vi "Test Sequence.vi"(0 "FeedBack Channel":string[](array[string])=["fgdgfvcbc", "vnfhgjkn", "21354682"], 1 "Test Name":string, 2 "Steps":T1(array[cluster]), 3 "Tracibility":bool) -> (6 "Emergency":bool, 7 "Out":i32, 8 "Condition":bool)   [LabVIEW 2015]
uses:
  <vilib>/Utility/error.llb/whitespace.ctl
  Galobal variable_TI.vi
  Project Setup/Globle Variable/GR_Servo.vi
  <vilib>/Instr/_visa.llb/VISA Configure Serial Port (Instr).vi
panel:
  out "error out 2":errorcluster
  out "error out":errorcluster
  out "Wait/Poll (ms)":u32
  out "Channels (Out)":i32[](array[numeric])
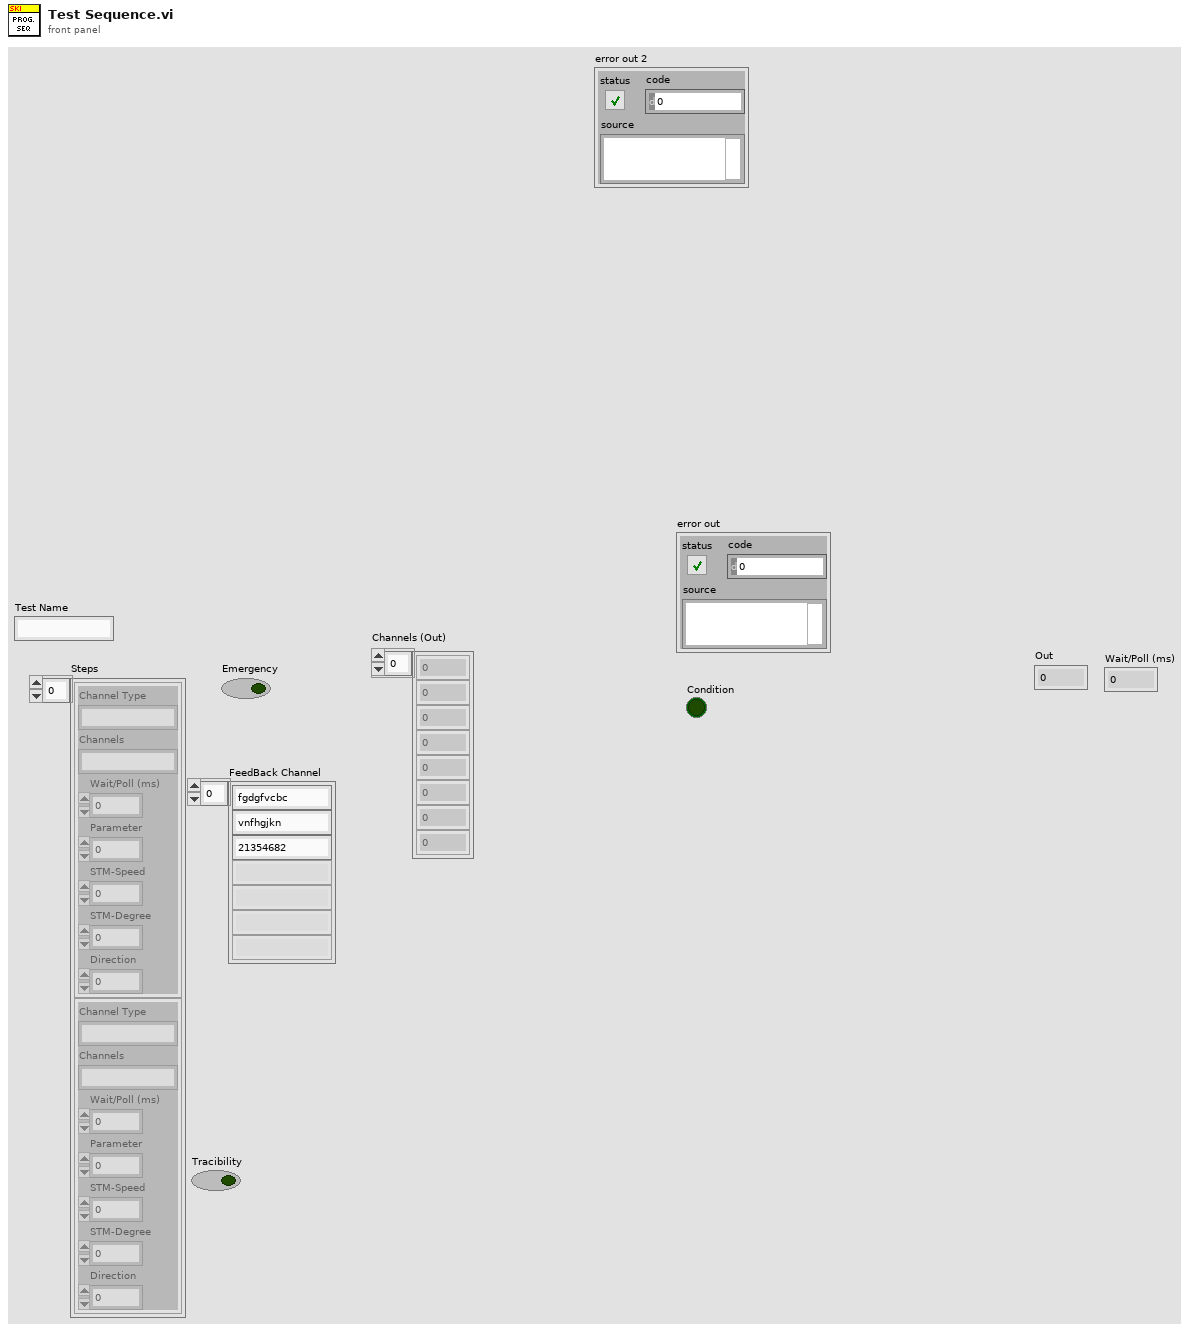
[diagram p1: front panel]
types:
  T1 = cluster{"Channel Type":string, "Channels":string, "Wait/Poll (ms)":u32, "Parameter":u8, "STM-Speed":i32, "STM-Degree":u32, "Direction":u8}[]
  T2 = cluster{"Emergency_1":bool, "Reset_2":bool, "Air Pressure_4":bool, "Safety Sensor_5":bool, "Safety Sensor_6":bool, "Barcode Rev rs_24":bool, "Clamp fwd rs_21":bool, "Servo Fault":bool, "Home _3":bool}
  T3 = cluster{"MIC ":refnum<visa-resource-name>, "baud rate MIC ":u32, "LCD ":refnum<visa-resource-name>, "baud rate_LCD":u32}
  T4 = cluster{"Model":string, "Difusser Code":string, "TFT Code ":string}
  T5 = typedef "whitespace.ctl" = u16
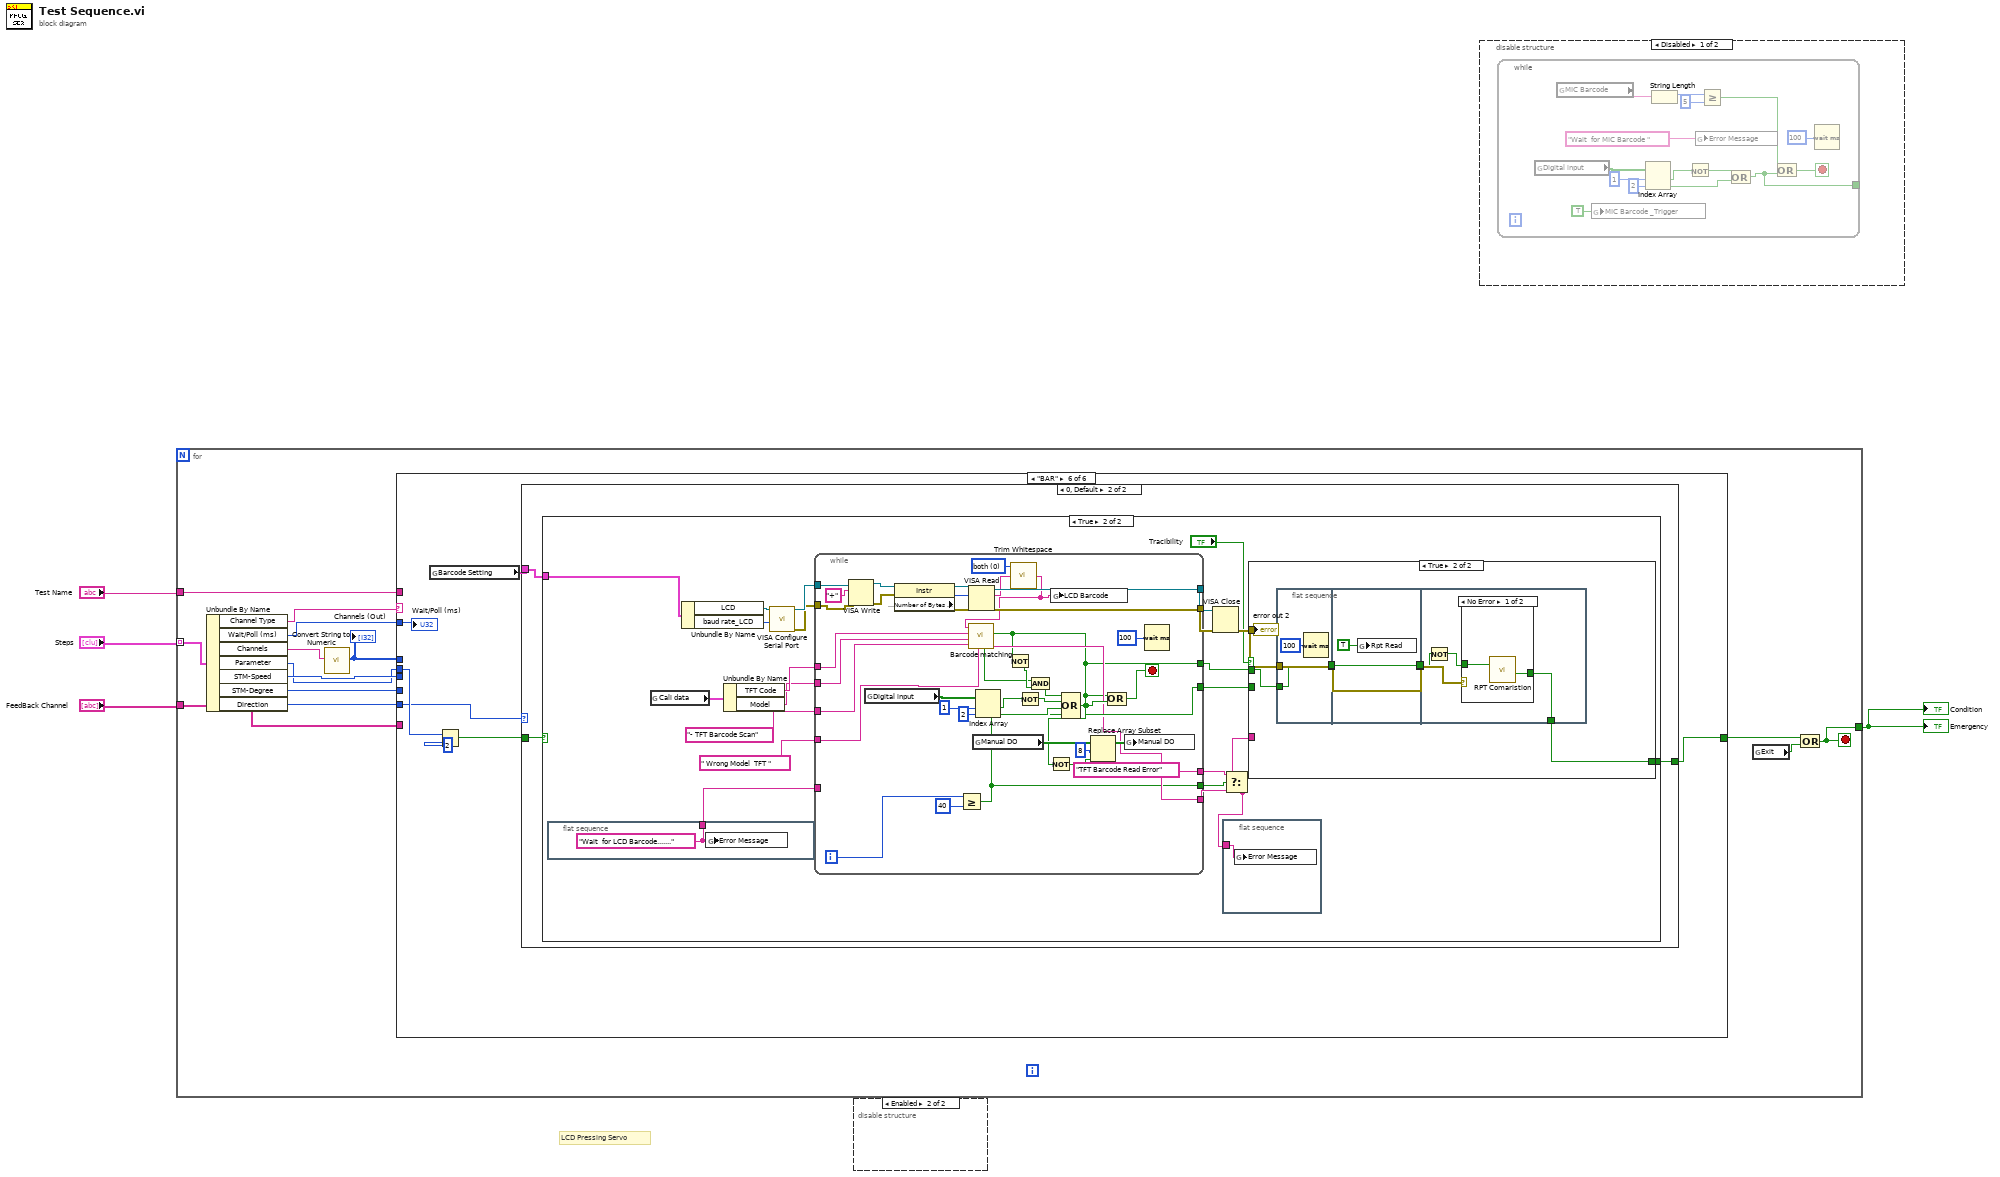
[diagram p0: block diagram]
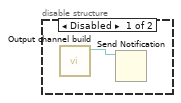
[diagram p3: hidden frame]
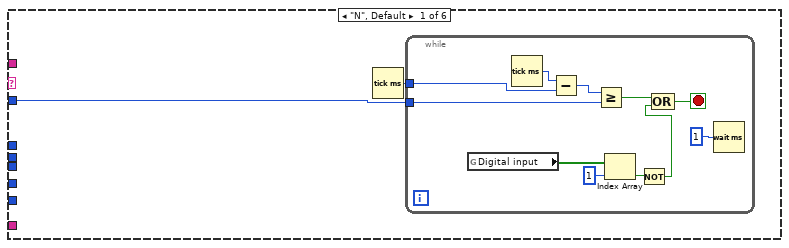
[diagram p4: hidden frame]
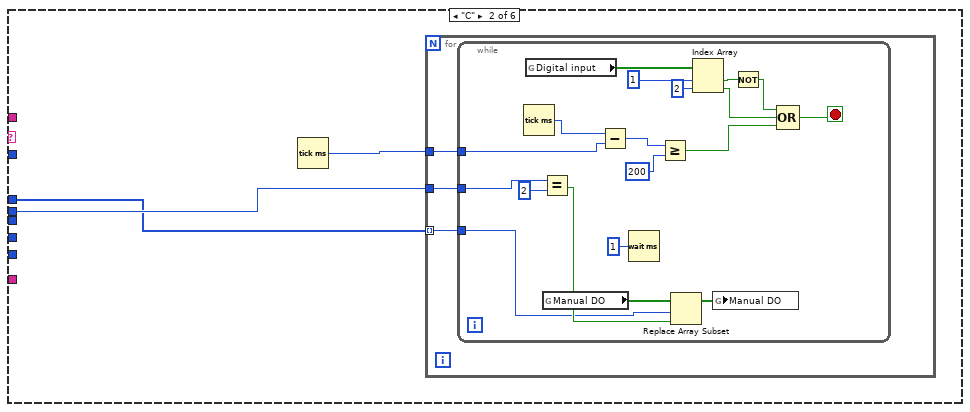
[diagram p5: hidden frame]
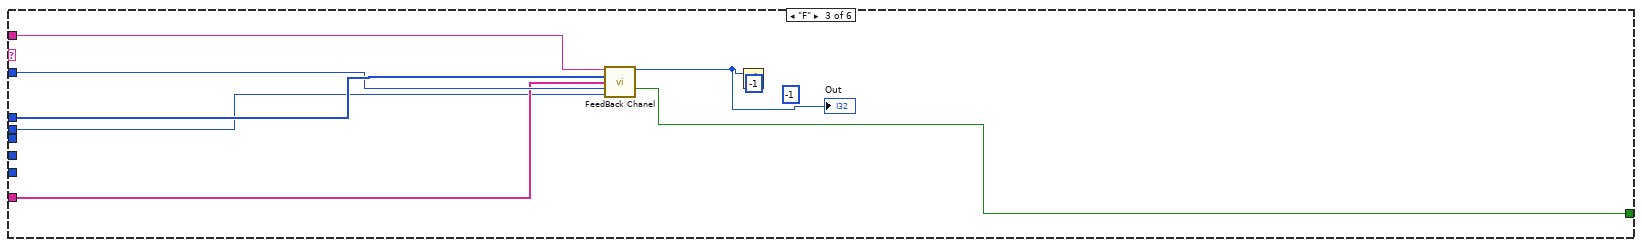
[diagram p6: hidden frame]
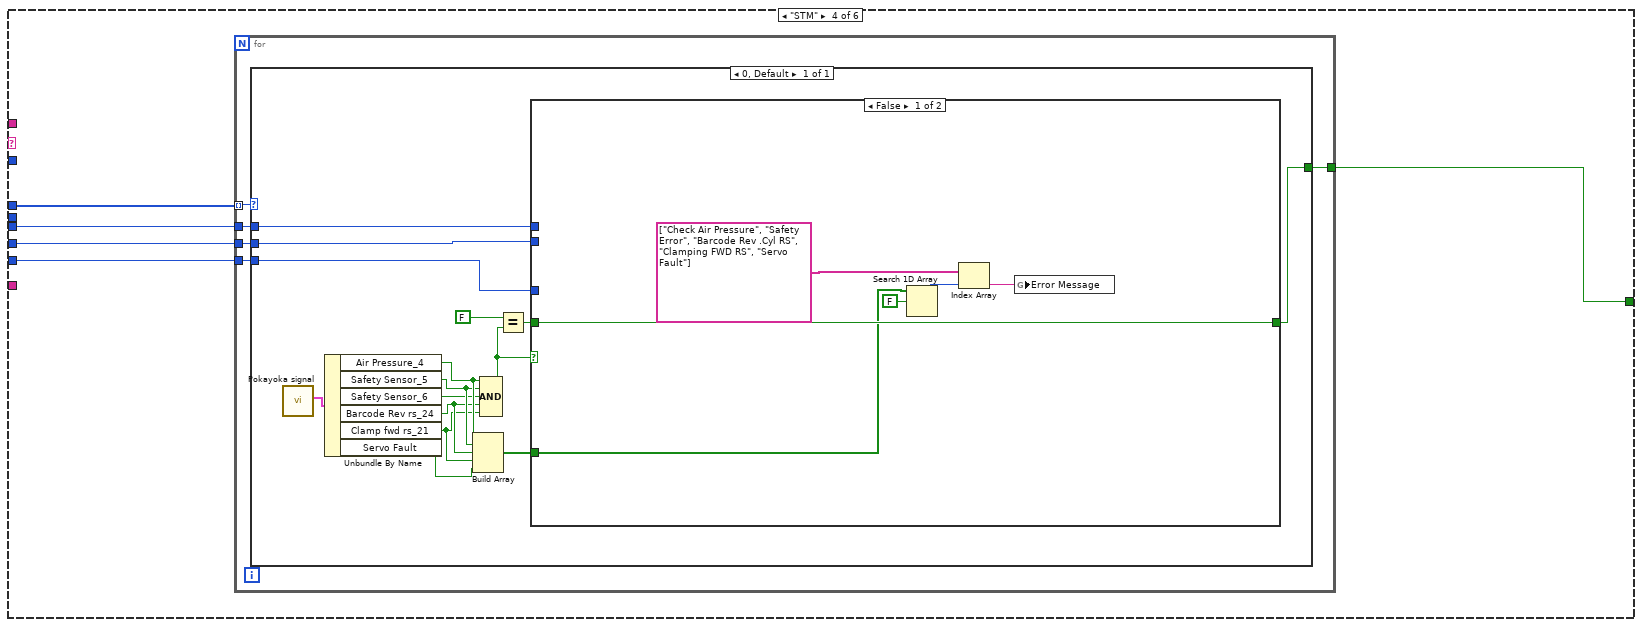
[diagram p7: hidden frame]
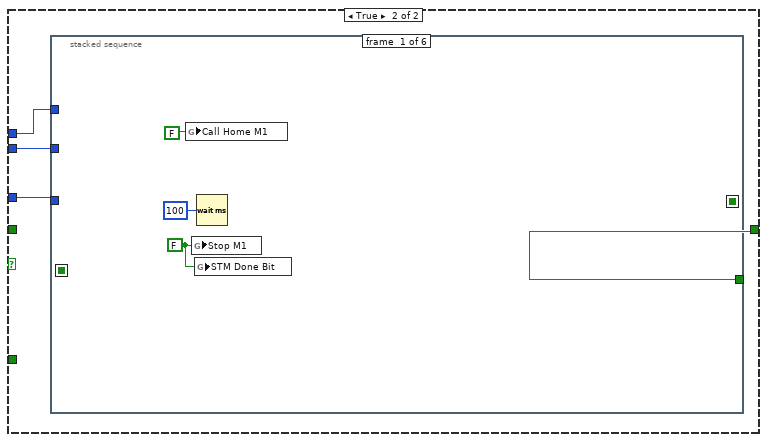
[diagram p8: hidden frame]
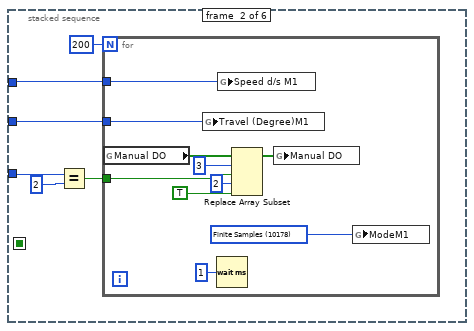
[diagram p9: hidden frame]
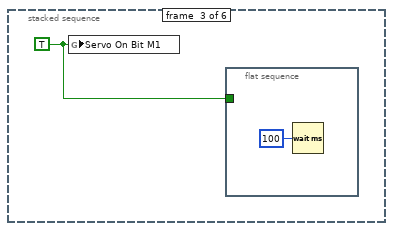
[diagram p10: hidden frame]
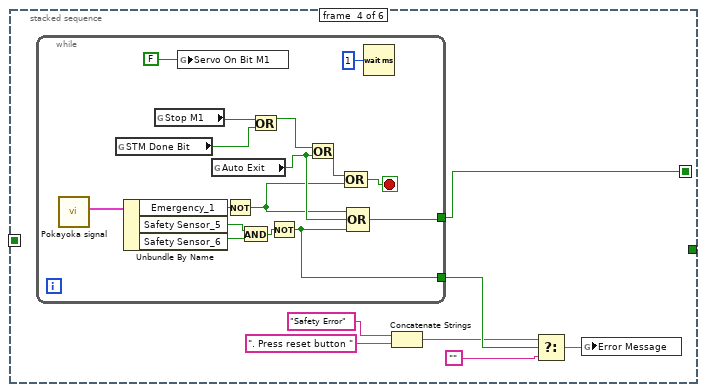
[diagram p11: hidden frame]
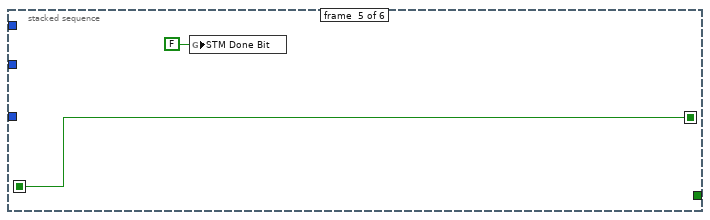
[diagram p12: hidden frame]
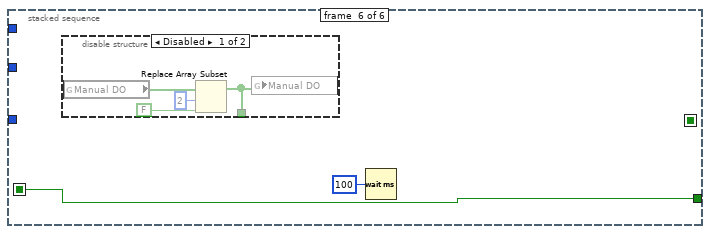
[diagram p13: hidden frame]
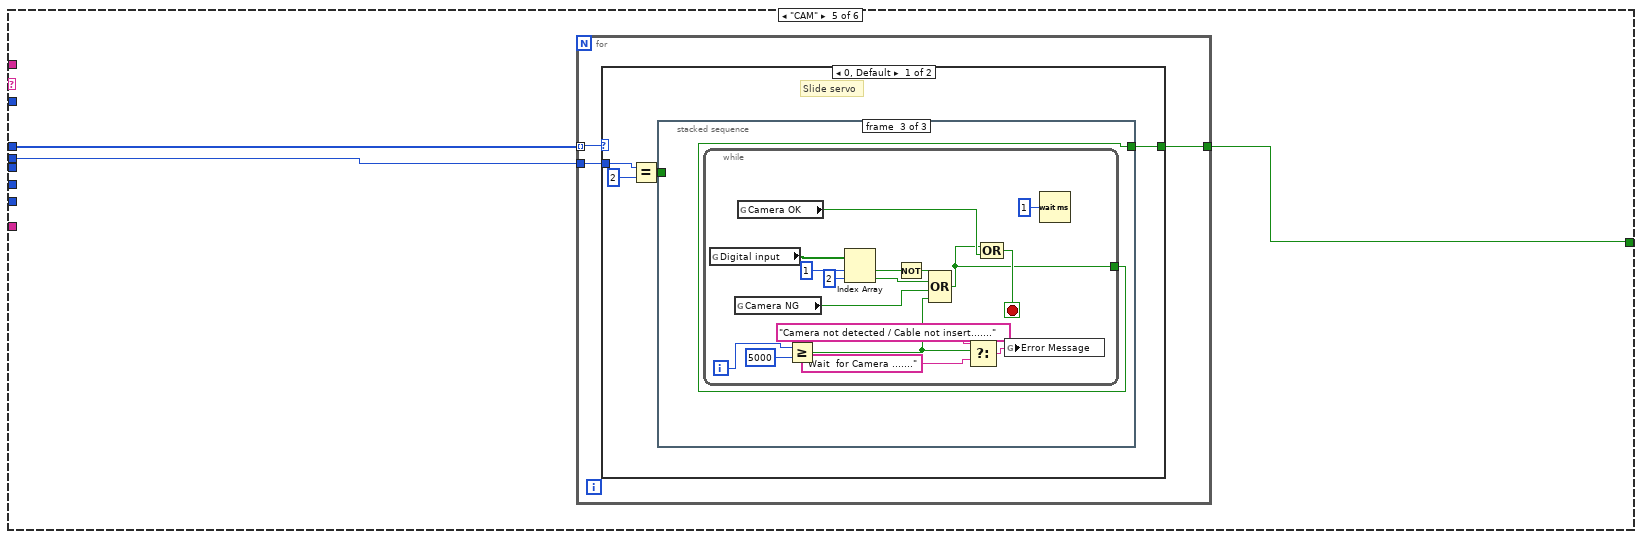
[diagram p15: hidden frame]
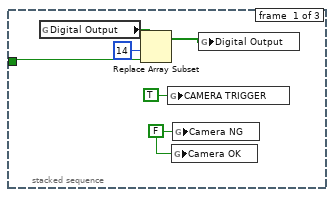
[diagram p16: hidden frame]
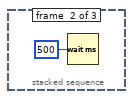
[diagram p17: hidden frame]
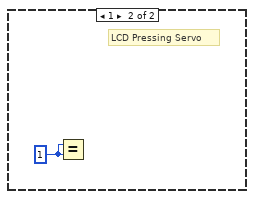
[diagram p18: hidden frame]
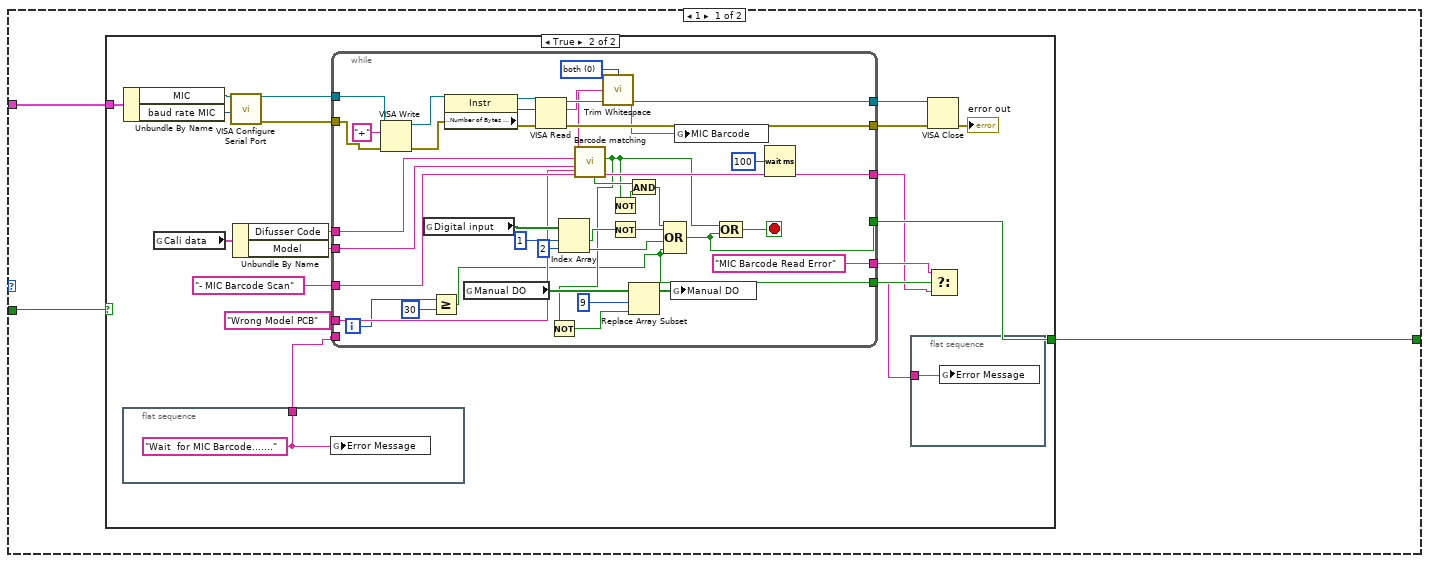
[diagram p19: hidden frame]
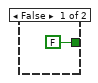
[diagram p20: hidden frame]
diagram:
  # "LCD Pressing Servo"
  n1 = for {
    tunnel: "Steps" -> [w18] mode=indexing
    tunnel: [w5] -> w1
    tunnel: "Test Name" -> [w13]
    tunnel: "FeedBack Channel" -> [w12]
    stop <- w5 stop-if-true
    n2 = Unbundle By Name(w18) -> ("Channel Type"=w17:string, "Wait/Poll (ms)"=w16:u32, "Channels"=w15:string, "Parameter"=w6:u8, "STM-Speed"=w8:i32, "STM-Degree"=w7:u32, "Direction"=w9:u8)
    n3 = call "Convert String to Numeric.vi"("Channels (A:B:C:D...) (In)"=w15) -> ("Channels (Out)"=w14:i32[])  [unwired: 9 in, 1 out]
    "Channels (Out)" <- w14
    n4 = case shown="\"BAR\"" w17 {
      tunnel: w16 -> [w19 _ w63 _ _ w194]
      tunnel: w14 -> [_ w32 w64 w69 w154 _]
      tunnel: w9 -> [_ _ _ w68 _ w189]
      tunnel: w13 -> [_ _ w62 _ _ _]
      tunnel: w12 -> [_ _ w61 _ _ _]
      tunnel: [_ _ w59 w65 w152 w190] -> w10
      tunnel: w8 -> [_ _ _ w67 _ _]
      tunnel: w7 -> [_ _ _ w66 _ _]
      tunnel: w6 -> [_ w34 w60 _ w153 w193]
      frame "N", Default {
        n5 = Tick Count (ms)() -> (millisecond timer value=w20:u32)
        n6 = while {
          tunnel: w20 -> [w30]
          tunnel: w19 -> [w25]
          stop <- w26 stop-if-true
          n7 = global read "Galobal variable_TI.vi" "Digital input"() -> (w24:bool[])
          n8 = Tick Count (ms)() -> (millisecond timer value=w31:u32)
          n9 = Subtract(x=w31, y=w30) -> (x-y=w29:u32)
          n10 = Greater Or Equal?(x=w29, y=w25) -> (x >= y?=w27:bool)
          n11 = Index Array(array=w24, index=1) -> (element=w22:bool)
          n12 = Not(x=w22) -> (.not. x?=w21:bool)
          n13 = Compound Arithmetic op=OR(w27, w21) -> (w26:bool)
          n14 = Wait (ms)(milliseconds to wait=u32 1) -> ()  [unwired: 1 out]
        }
      }
      frame "C" {
        n15 = Tick Count (ms)() -> (millisecond timer value=w33:u32)
        n16 = for {
          tunnel: w32 -> [w36] mode=indexing
          tunnel: w34 -> [w37]
          tunnel: w33 -> [w35]
          n17 = while {
            tunnel: w37 -> [w56]
            tunnel: w36 -> [w50]
            tunnel: w35 -> [w48]
            stop <- w44 stop-if-true
            n18 = Tick Count (ms)() -> (millisecond timer value=w49:u32)
            n19 = global read "Galobal variable_TI.vi" "Digital input"() -> (w43:bool[])
            n20 = Equal?(x=w56, y=u8 2) -> (x = y?=w51:bool)
            n21 = global read "Galobal variable_TI.vi" "Manual DO"() -> (w52:bool[])
            n22 = Subtract(x=w49, y=w48) -> (x-y=w47:u32)
            n23 = Wait (ms)(milliseconds to wait=u32 1) -> ()  [unwired: 1 out]
            n24 = Greater Or Equal?(x=w47, y=u32 200) -> (x >= y?=w45:bool)
            n25 = Replace Array Subset(array=w52, new element=w51, index=w50) -> (w53:bool[])
            n26 = Index Array(array=w43, index #1=1 ("index"), index #2=2 ("index")) -> (element #1=w41:bool, element #2=w38:bool)
            n27 = global write "Galobal variable_TI.vi" "Manual DO"(w53) -> ()
            n28 = Not(x=w41) -> (.not. x?=w39:bool)
            n29 = Compound Arithmetic op=OR(w39, w38, w45) -> (w44:bool)
          }
        }
      }
      frame "F" {
        (unwired) -1 ("Out")
        n30 = call "FeedBack Chanel.vi"("Test Name"=w62, "Channels (Int)"=w64, "FeedBack Channel"=w61, "Wait/Poll (ms)"=w63, "Parameter"=w60) -> ("Out"=w57:i32, "Fail"=w59:bool)  [unwired: 6 in, 3 out]
        "Out" <- w57
        n31 = Not Equal?(x=w57, y=-1) -> ()  [unwired: 1 out]
      }
      frame "STM" {
        n32 = for {
          tunnel: w69 -> [w74] mode=indexing
          tunnel: w68 -> [w73]
          tunnel: w67 -> [w72]
          tunnel: w66 -> [w71]
          tunnel: [w70] -> w65
          n33 = case shown="0, Default" w74 {
            tunnel: w73 -> [w87]
            tunnel: w72 -> [w89]
            tunnel: w71 -> [w88]
            tunnel: [w84] -> w70
            frame 0, Default {
              n34 = call "Pokayoka signal.vi"() -> ("output cluster"=w83:T2)  [unwired: 10 in, 1 out]
              n35 = Unbundle By Name(w83) -> ("Air Pressure_4"=w81:bool, "Safety Sensor_5"=w80:bool, "Safety Sensor_6"=w79:bool, "Barcode Rev rs_24"=w77:bool, "Clamp fwd rs_21"=w76:bool, "Servo Fault"=w75:bool)
              n36 = Build Array(w81, w80, w77, w76, w75) -> (w78:bool[])
              n37 = Compound Arithmetic op=AND(w81, w80, w79, w77, w76) -> (w82:bool)
              n38 = Equal?(x=FALSE ("y"), y=w82) -> (x = y?=w85:bool)
              n39 = case shown="False" w82 {
                tunnel: w89 -> [_ w99]
                tunnel: w88 -> [_ w98]
                tunnel: w87 -> [_ w97]
                tunnel: [w95 w96] -> w84
                tunnel: w85 -> [w95 _]
                tunnel: w78 -> [w94 _]
                frame False {
                  n40 = Search 1D Array(1D array=w94, element=FALSE) -> (index of element=w91:i32)  [unwired: 1 in]
                  n41 = Index Array(array=string[] ["Check Air Pressure", "Safety Error", "Barcode Rev .Cyl RS", "Clamping FWD RS", "Servo Fault"], index=w91) -> (element=w90:string)
                  n42 = global write "GR_Servo.vi" "Error Message"(w90) -> ()
                }
                frame True {
                  n43 = stacked-sequence {
                    seq-local: [_ _ _ w127 _ _] -> [_ _ _ _ w144 _]
                    seq-local: [_ _ _ _ w144 _] -> [_ _ _ _ _ w146]
                    tunnel: w98 -> [_ w108 _ _ _ _]
                    tunnel: w97 -> [_ w106 _ _ _ _]
                    tunnel: w99 -> [_ w104 _ _ _ _]
                    tunnel: [_ _ _ _ _ w146] -> w96
                    frame #0 {
                      w100 = FALSE ("Stop M1")
                      n44 = global write "Galobal variable_TI.vi" "Call Home M1"(FALSE ("Call Home M2")) -> ()
                      n45 = global write "Galobal variable_TI.vi" "Stop M1"(w100) -> ()
                      n46 = global write "Galobal variable_TI.vi" "STM Done Bit"(w100) -> ()
                      n47 = Wait (ms)(milliseconds to wait=u32 100) -> ()  [unwired: 1 out]
                    }
                    frame #1 {
                      n48 = Equal?(x=w106, y=u8 2) -> (x = y?=w105:bool)
                      n49 = for {
                        N: 200 -> [_]
                        tunnel: w108 -> [w118]
                        tunnel: w105 -> [w116]
                        tunnel: w104 -> [w114]
                        w117 = 10178 items=["Finite Samples"=10178, "Continuous Samples"=10123, "Hardware Timed Single Point"=12522] ("ModeM1")
                        n50 = global read "Galobal variable_TI.vi" "Manual DO"() -> (w112:bool[])
                        n51 = global write "GR_Servo.vi" "Travel (Degree)M1"(w118) -> ()
                        n52 = Wait (ms)(milliseconds to wait=u32 1) -> ()  [unwired: 1 out]
                        n53 = global write "GR_Servo.vi" "Speed d/s M1"(w114) -> ()
                        n54 = Replace Array Subset(array=w112, new element #1=w116, index #1=3 ("index"), new element #2=TRUE ("new element/subarray"), index #2=2 ("index")) -> (w115:bool[])
                        n55 = global write "Galobal variable_TI.vi" "Manual DO"(w115) -> ()
                        n56 = global write "GR_Servo.vi" "ModeM1"(w117) -> ()
                      }
                    }
                    frame #2 {
                      w119 = TRUE ("Servo On Bit")
                      n57 = global write "GR_Servo.vi" "Servo On Bit M1"(w119) -> ()
                      n58 = flat-sequence {
                        tunnel: w119 -> [_]
                        frame #0 {
                          n59 = Wait (ms)(milliseconds to wait=u32 100) -> ()  [unwired: 1 out]
                        }
                      }
                    }
                    frame #3 {
                      n60 = while {
                        tunnel: [w133] -> w127
                        tunnel: [w128] -> w125
                        stop <- w136 stop-if-true
                        n61 = call "Pokayoka signal.vi"() -> ("output cluster"=w138:T2)  [unwired: 10 in, 1 out]
                        n62 = global read "Galobal variable_TI.vi" "STM Done Bit"() -> (w141:bool)
                        n63 = Unbundle By Name(w138) -> ("Emergency_1"=w135:bool, "Safety Sensor_5"=w131:bool, "Safety Sensor_6"=w130:bool)
                        n64 = global read "Galobal variable_TI.vi" "Stop M1"() -> (w142:bool)
                        n65 = global write "GR_Servo.vi" "Servo On Bit M1"(FALSE ("Servo On Bit")) -> ()
                        n66 = global read "Galobal variable_TI.vi" "Auto Exit"() -> (w134:bool)
                        n67 = Not(x=w135) -> (.not. x?=w132:bool)
                        n68 = And(x=w131, y=w130) -> (x .and. y?=w129:bool)
                        n69 = Or(x=w142, y=w141) -> (x .or. y?=w139:bool)
                        n70 = Not(x=w129) -> (.not. x?=w128:bool)
                        n71 = Or(x=w139, y=w134) -> (x .or. y?=w137:bool)
                        n72 = Compound Arithmetic op=OR(w137, w132) -> (w136:bool)
                        n73 = Compound Arithmetic op=OR(w132, w134, w128) -> (w133:bool)
                        n74 = Wait (ms)(milliseconds to wait=u32 1) -> ()  [unwired: 1 out]
                      }
                      n75 = Concatenate Strings("Safety Error" ("string"), ". Press reset button ") -> (w123:string)
                      n76 = Select(t=w123, s=w125, f="") -> (s? t:f=w126:string)
                      n77 = global write "GR_Servo.vi" "Error Message"(w126) -> ()
                    }
                    frame #4 {
                      n78 = global write "Galobal variable_TI.vi" "STM Done Bit"(FALSE ("STM Done Bit LCD Pressing")) -> ()
                    }
                    frame #5 {
                      n79 = disable-structure shown="Disabled" {
                        disable-tunnel: [w148 _] -> _
                        frame Disabled {
                          n80 = global read "Galobal variable_TI.vi" "Manual DO"() -> (w151:bool[])
                          n81 = Replace Array Subset(array=w151, new element=FALSE ("new element/subarray"), index=2) -> (w148:bool[])
                          n82 = global write "Galobal variable_TI.vi" "Manual DO"(w148) -> ()
                        }
                        frame Enabled {
                        }
                      }
                      n83 = Wait (ms)(milliseconds to wait=u32 100) -> ()  [unwired: 1 out]
                    }
                  }
                }
              }
            }
          }
        }
      }
      frame "CAM" {
        n84 = for {
          tunnel: w154 -> [w157] mode=indexing
          tunnel: w153 -> [w156]
          tunnel: [w155] -> w152
          n85 = case shown="0, Default" w157 {
            tunnel: w156 -> [w161 _]
            tunnel: [w158 _] -> w155
            frame 0, Default {
              # "Slide servo"
              n86 = Equal?(x=w161, y=u8 2) -> (x = y?=w159:bool)
              n87 = stacked-sequence {
                tunnel: w159 -> [w166 _ _]
                tunnel: [_ _ w169] -> w158
                frame #0 {
                  w162 = FALSE ("Camera NG")
                  n88 = global read "Galobal variable_TI.vi" "Digital Output"() -> (w167:bool[])
                  n89 = Replace Array Subset(array=w167, new element=w166, index=14) -> (w165:bool[])
                  n90 = global write "Galobal variable_TI.vi" "CAMERA TRIGGER"(TRUE ("CAMERA TRIGGER")) -> ()
                  n91 = global write "Galobal variable_TI.vi" "Camera OK"(w162) -> ()
                  n92 = global write "Galobal variable_TI.vi" "Camera NG"(w162) -> ()
                  n93 = global write "Galobal variable_TI.vi" "Digital Output"(w165) -> ()
                }
                frame #1 {
                  n94 = Wait (ms)(milliseconds to wait=u32 500) -> ()  [unwired: 1 out]
                }
                frame #2 {
                  n95 = while {
                    tunnel: [w177] -> w169
                    i -> [w175]
                    stop <- w178 stop-if-true
                    n96 = global read "Galobal variable_TI.vi" "Digital input"() -> (w185:bool[])
                    n97 = global read "Galobal variable_TI.vi" "Camera NG"() -> (w180:bool)
                    n98 = global read "Galobal variable_TI.vi" "Camera OK"() -> (w179:bool)
                    n99 = Greater Or Equal?(x=w175, y=5000) -> (x >= y?=w173:bool)
                    n100 = Index Array(array=w185, index #1=1 ("index"), index #2=2 ("index")) -> (element #1=w182:bool, element #2=w186:bool)
                    n101 = Not(x=w182) -> (.not. x?=w181:bool)
                    n102 = Compound Arithmetic op=OR(w181, w186, w180, w173) -> (w177:bool)
                    n103 = Select(t="Camera not detected / Cable not insert.......", s=w173, f="Wait  for Camera .......") -> (s? t:f=w172:string)
                    n104 = Compound Arithmetic op=OR(w177, w179) -> (w178:bool)
                    n105 = global write "GR_Servo.vi" "Error Message"(w172) -> ()
                    n106 = Wait (ms)(milliseconds to wait=u32 1) -> ()  [unwired: 1 out]
                  }
                }
              }
            }
            frame 1 {
              w187 = u8 1 ("y")
              # "LCD Pressing Servo"
              n107 = Equal?(x=w187, y=w187) -> ()  [unwired: 1 out]
            }
          }
        }
      }
      frame "BAR" {
        n108 = global read "Galobal variable_TI.vi" "Barcode Setting"() -> (w188:T3)
        n109 = Equal?(x=w193, y=u8 2) -> (x = y?=w191:bool)
        n110 = case shown="0, Default" w189 {
          tunnel: w191 -> [w197 w261]
          tunnel: w188 -> [w196 w260]
          tunnel: [w195 w259] -> w190
          frame 1 {
            n111 = case shown="True" w197 {
              tunnel: w196 -> [_ w217]
              tunnel: [FALSE w209] -> w195
              frame False {
              }
              frame True {
                n112 = flat-sequence {
                  tunnel: [w219] -> w203
                  frame #0 {
                    w219 = "Wait  for MIC Barcode......."
                    n113 = global write "GR_Servo.vi" "Error Message"(w219) -> ()
                  }
                }
                n114 = Unbundle By Name(w217) -> ("MIC"=w216:refnum<visa-resource-name>, "baud rate MIC"=w215:u32)
                n115 = global read "Galobal variable_TI.vi" "Cali data"() -> (w208:T4)
                n116 = call-poly "VISA Configure Serial Port"("VISA resource name"=w216, "baud rate (9600)"=w215) -> ("VISA resource name out"=w214:refnum<visa-resource-name>, "error out"=w213:errorcluster)  [unwired: 12 in]
                n117 = Unbundle By Name(w208) -> ("Difusser Code"=w207:string, "Model"=w206:string)
                n118 = while {
                  tunnel: w214 -> [w238]
                  tunnel: w213 -> [w236]
                  tunnel: [w255] -> w212
                  tunnel: [w254] -> w211
                  tunnel: [w232] -> w209
                  tunnel: w207 -> [w242]
                  tunnel: w206 -> [w241]
                  tunnel: "- MIC Barcode Scan" ("TFT BARCODE SCANE") -> [w240]
                  tunnel: "Wrong Model PCB" ("TFT WORNG SCANE") -> [w239]
                  tunnel: w203 -> [_]
                  tunnel: [w231] -> w200
                  tunnel: [w224] -> w202
                  tunnel: ["MIC Barcode Read Error"] -> w201
                  i -> [w225]
                  stop <- w233 stop-if-true
                  w222 = T5 0 items=["both", "start of string", "end of string"] ("location (both)")
                  n119 = VISA Write(VISA resource name=w238, write buffer="+", error in (no error)=w236) -> (VISA resource name out=w237:refnum<visa-resource-name>, error out=w235:errorcluster)  [unwired: 1 out]
                  n120 = global read "Galobal variable_TI.vi" "Digital input"() -> (w253:bool[])
                  n121 = Greater Or Equal?(x=w225, y=30) -> (x >= y?=w224:bool)
                  n122 = property class="Instr"(reference=w237, error in=w235) -> (reference out=w258:refnum<visa-resource-name>, error out=w257:errorcluster, "Serial Settings:Number of Bytes at Serial Port"=w256:u32)
                  n123 = global read "Galobal variable_TI.vi" "Manual DO"() -> (w245:bool[])
                  n124 = VISA Read(VISA resource name=w258, byte count=w256, error in (no error)=w257) -> (VISA resource name out=w255:refnum<visa-resource-name>, read buffer=w221:string, error out=w254:errorcluster)  [unwired: 1 out]
                  n125 = Index Array(array=w253, index #1=1 ("index"), index #2=2 ("index")) -> (element #1=w250:bool, element #2=w248:bool)
                  n126 = call <vilib>:"Trim Whitespace.vi"("string"=w221, "location (both)"=w222) -> ("trimmed string"=w220:string)
                  n127 = call "Barcode matching.vi"("TFT WORNG SCANE"=w239, "TFT BARCODE SCANE"=w240, "Model"=w241, "TFT Code"=w242, "Serial data"=w220) -> ("Error"=w231:string, "result/trigger"=w229:bool, "Read bit"=w230:bool)  [unwired: 2 in, 2 out]
                  n128 = Not(x=w229) -> (.not. x?=w243:bool)
                  n129 = Not(x=w229) -> (.not. x?=w228:bool)
                  n130 = Not(x=w250) -> (.not. x?=w249:bool)
                  n131 = And(x=w230, y=w228) -> (x .and. y?=w227:bool)
                  n132 = Replace Array Subset(array=w245, new element=w243, index=9) -> (w246:bool[])
                  n133 = Compound Arithmetic op=OR(w227, w249, w248, w224) -> (w232:bool)
                  n134 = global write "Galobal variable_TI.vi" "Manual DO"(w246) -> ()
                  n135 = global write "Galobal variable_TI.vi" "MIC Barcode"(w220) -> ()
                  n136 = Compound Arithmetic op=OR(w229, w232) -> (w233:bool)
                  n137 = Wait (ms)(milliseconds to wait=u32 100) -> ()  [unwired: 1 out]
                }
                n138 = flat-sequence {
                  tunnel: w199 -> [w218]
                  frame #0 {
                    n139 = global write "GR_Servo.vi" "Error Message"(w218) -> ()
                  }
                }
                n140 = VISA Close(VISA resource name=w212, error in (no error)=w211) -> (error out=→"error out":errorcluster)
                n141 = Select(t=w201, s=w202, f=w200) -> (s? t:f=w199:string)
              }
            }
          }
          frame 0, Default {
            n142 = case shown="True" w261 {
              tunnel: w260 -> [_ w284]
              tunnel: [FALSE w266] -> w259
              frame False {
                # "barcode bypass"
              }
              frame True {
                n143 = flat-sequence {
                  tunnel: [w306] -> w272
                  frame #0 {
                    w306 = "Wait  for LCD Barcode......."
                    n144 = global write "GR_Servo.vi" "Error Message"(w306) -> ()
                  }
                }
                n145 = global read "Galobal variable_TI.vi" "Cali data"() -> (w277:T4)
                n146 = Unbundle By Name(w284) -> ("LCD"=w283:refnum<visa-resource-name>, "baud rate_LCD"=w282:u32)
                n147 = Unbundle By Name(w277) -> ("TFT Code"=w276:string, "Model"=w275:string)
                n148 = call-poly "VISA Configure Serial Port"("VISA resource name"=w283, "baud rate (9600)"=w282) -> ("VISA resource name out"=w281:refnum<visa-resource-name>, "error out"=w280:errorcluster)  [unwired: 12 in]
                n149 = while {
                  tunnel: w281 -> [w324]
                  tunnel: w280 -> [w323]
                  tunnel: [w342] -> w279
                  tunnel: [w341] -> w278
                  tunnel: [w319] -> w264
                  tunnel: w276 -> [w329]
                  tunnel: w275 -> [w328]
                  tunnel: "- TFT Barcode Scan" ("TFT BARCODE SCANE") -> [w327]
                  tunnel: " Wrong Model  TFT " ("TFT WORNG SCANE") -> [w326]
                  tunnel: w272 -> [_]
                  tunnel: [w318] -> w269
                  tunnel: [w312] -> w271
                  tunnel: ["TFT Barcode Read Error"] -> w270
                  tunnel: [w310] -> w267
                  i -> [w313]
                  stop <- w320 stop-if-true
                  w308 = T5 0 items=["both", "start of string", "end of string"] ("location (both)")
                  n150 = VISA Write(VISA resource name=w324, write buffer="+", error in (no error)=w323) -> (VISA resource name out=w322:refnum<visa-resource-name>, error out=w321:errorcluster)  [unwired: 1 out]
                  n151 = global read "Galobal variable_TI.vi" "Digital input"() -> (w340:bool[])
                  n152 = property class="Instr"(reference=w322, error in=w321) -> (reference out=w345:refnum<visa-resource-name>, error out=w344:errorcluster, "Serial Settings:Number of Bytes at Serial Port"=w343:u32)
                  n153 = Greater Or Equal?(x=w313, y=40) -> (x >= y?=w312:bool)
                  n154 = VISA Read(VISA resource name=w345, byte count=w343, error in (no error)=w344) -> (VISA resource name out=w342:refnum<visa-resource-name>, read buffer=w309:string, error out=w341:errorcluster)  [unwired: 1 out]
                  n155 = global read "Galobal variable_TI.vi" "Manual DO"() -> (w332:bool[])
                  n156 = Index Array(array=w340, index #1=1 ("index"), index #2=2 ("index")) -> (element #1=w337:bool, element #2=w335:bool)
                  n157 = call <vilib>:"Trim Whitespace.vi"("string"=w309, "location (both)"=w308) -> ("trimmed string"=w307:string)
                  n158 = call "Barcode matching.vi"("TFT WORNG SCANE"=w326, "TFT BARCODE SCANE"=w327, "Model"=w328, "TFT Code"=w329, "Serial data"=w307) -> ("Error"=w318:string, "result/trigger"=w310:bool, "Read bit"=w316:bool)  [unwired: 2 in, 2 out]
                  n159 = Not(x=w310) -> (.not. x?=w317:bool)
                  n160 = Not(x=w337) -> (.not. x?=w336:bool)
                  n161 = And(x=w316, y=w317) -> (x .and. y?=w315:bool)
                  n162 = Not(x=w310) -> (.not. x?=w331:bool)
                  n163 = global write "Galobal variable_TI.vi" "LCD Barcode"(w307) -> ()
                  n164 = Compound Arithmetic op=OR(w315, w336, w335, w312) -> (w319:bool)
                  n165 = Replace Array Subset(array=w332, new element=w331, index=8) -> (w333:bool[])
                  n166 = Compound Arithmetic op=OR(w310, w319) -> (w320:bool)
                  n167 = global write "Galobal variable_TI.vi" "Manual DO"(w333) -> ()
                  n168 = Wait (ms)(milliseconds to wait=u32 100) -> ()  [unwired: 1 out]
                }
                n169 = VISA Close(VISA resource name=w279, error in (no error)=w278) -> (error out=w268:errorcluster)
                n170 = flat-sequence {
                  tunnel: w263 -> [w305]
                  frame #0 {
                    n171 = global write "GR_Servo.vi" "Error Message"(w305) -> ()
                  }
                }
                n172 = Select(t=w270, s=w271, f=w269) -> (s? t:f=w263:string)
                n173 = case shown="True" "Tracibility" {
                  tunnel: w268 -> [_ w288]
                  tunnel: w267 -> [_ w287]
                  tunnel: [w285 w286] -> w266
                  tunnel: w264 -> [w285 _]
                  tunnel: w263 -> [_ _]
                  frame False {
                  }
                  frame True {
                    n174 = flat-sequence {
                      tunnel: w287 -> [w294]
                      tunnel: w288 -> [w295]
                      tunnel: [w295] -> w292
                      tunnel: [w294] -> w291
                      tunnel: [w298] -> w290
                      tunnel: [w297] -> w289
                      tunnel: w292 -> [w298]
                      tunnel: w291 -> [w297]
                      tunnel: [w300] -> w286
                      tunnel: w290 -> [w302]
                      tunnel: w289 -> [w301]
                      frame #0 {
                        n175 = Wait (ms)(milliseconds to wait=u32 100) -> ()  [unwired: 1 out]
                      }
                      frame #1 {
                        n176 = global write "Galobal variable_TI.vi" "Rpt Read"(TRUE ("Rpt Read")) -> ()
                      }
                      frame #2 {
                        n177 = Not(x=w301) -> (.not. x?=w299:bool)
                        n178 = case shown="No Error" w302 {
                          tunnel: w299 -> [w304 _]
                          tunnel: [w303 _] -> w300
                          frame No Error {
                            n179 = call "RPT Comaristion.vi"("True"=w304) -> ("Fail"=w303:bool)  [unwired: 10 in]
                          }
                          frame Error {
                          }
                        }
                      }
                    }
                    "error out 2" <- w288
                  }
                }
              }
            }
          }
        }
        "Wait/Poll (ms)" <- w194
      }
    }
    n180 = global read "Galobal variable_TI.vi" "Exit"() -> (w11:bool)
    n181 = Compound Arithmetic op=OR(w10, w11) -> (w5:bool)
  }
  "Emergency" <- w1
  "Condition" <- w1
  n182 = disable-structure shown="Enabled" {
    frame Disabled {
      n183 = call "Output channel build.vi"() -> ("Output channel"=w346:refnum<notifier>)  [unwired: 11 in]
      n184 = Send Notification(notifier=w346) -> ()  [unwired: 2 in, 2 out]
    }
    frame Enabled {
    }
  }
  n185 = disable-structure shown="Disabled" {
    frame Disabled {
      n186 = while {
        tunnel: [w353] -> _
        stop <- w355 stop-if-true
        n187 = global read "Galobal variable_TI.vi" "Digital input"() -> (w361:bool[])
        n188 = global read "Galobal variable_TI.vi" "MIC Barcode"() -> (w352:string)
        n189 = global write "Galobal variable_TI.vi" "MIC Barcode _Trigger"(TRUE ("MIC Barcode _Trigger")) -> ()
        n190 = Index Array(array=w361, index #1=1 ("index"), index #2=2 ("index")) -> (element #1=w358:bool, element #2=w356:bool)
        n191 = String Length(string=w352) -> (length=w351:i32)
        n192 = Not(x=w358) -> (.not. x?=w357:bool)
        n193 = global write "GR_Servo.vi" "Error Message"("Wait  for MIC Barcode ") -> ()
        n194 = Greater Or Equal?(x=w351, y=5) -> (x >= y?=w349:bool)
        n195 = Compound Arithmetic op=OR(w357, w356) -> (w353:bool)
        n196 = Compound Arithmetic op=OR(w349, w353) -> (w355:bool)
        n197 = Wait (ms)(milliseconds to wait=u32 100) -> ()  [unwired: 1 out]
      }
    }
    frame Enabled {
    }
  }
